vi "Read Field properties.vi"(8 "error in (no error)":errorcluster, 11 "HC-ScanParser in":refnum<class "HC-ScanParser.lvclass">) -> (0 "error out":errorcluster, 2 "Field properties":T1={"Layer height"=0.05000000074505806, "MaximumFieldWidth"=0.0, "MaximumFieldHeight"=0.0, "MaximumFieldRadius"=40.0, "MaxAcceleration"=10000000.0, "MaxMarkSpeed"=10000.0, "MaxJumpSpeed"=10000.0}, 3 "HC-ScanParser out":refnum<class "HC-ScanParser.lvclass">)   [LabVIEW 2013, in "HardwareCharacterization.lvlib" / "HC-ScanParser.lvclass"]
uses:
  HC-ScanParser.lvclass
  Field-properties.ctl
  HC-ScanParser.lvclass/HC-ScanParser.ctl
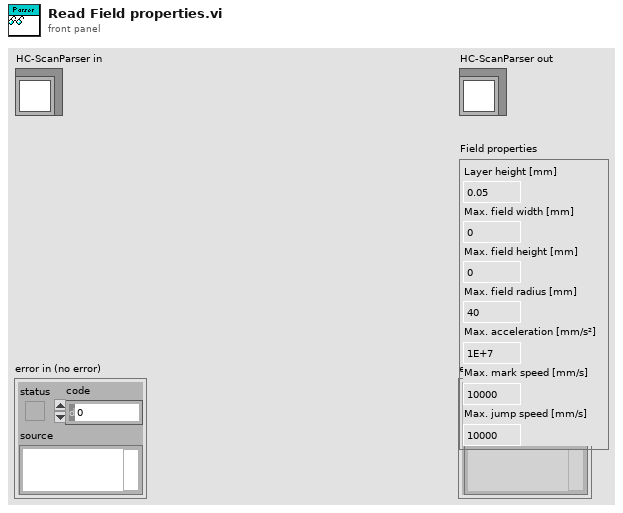
[diagram p1: front panel]
types:
  T1 = typedef "HardwareCharacterization.lvlib/HC-ScanParser.lvclass/Field-properties.ctl" = cluster{"Layer height":dbl, "MaximumFieldWidth":dbl, "MaximumFieldHeight":dbl, "MaximumFieldRadius":dbl, "MaxAcceleration":dbl, "MaxMarkSpeed":dbl, "MaxJumpSpeed":dbl}
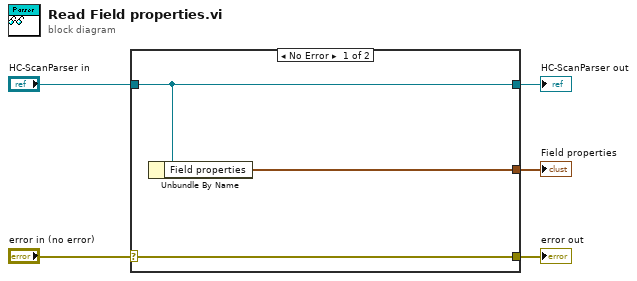
[diagram p0: block diagram]
diagram:
  n1 = case shown="No Error" "error in (no error)" {
    selector: "error in (no error)" -> [w8 w9]
    tunnel: [w8 w9] -> w4
    tunnel: [w7 w10] -> w2
    tunnel: "HC-ScanParser in" -> [w7 w10]
    tunnel: [w6 _] -> w1
    frame No Error {
      n2 = Unbundle By Name(w7) -> ("Field properties"=w6:T1)
    }
    frame Error {
    }
  }
  "error out" <- w4
  "HC-ScanParser out" <- w2
  "Field properties" <- w1
